vi "Compute Optimal Transition Time.vi"(8 "error in (no error)":errorcluster, 10 "optimum":T1, 11 "SV Square in":refnum<class "SV Square.lvclass">) -> (0 "error out":errorcluster, 2 "optimal transition time":dbl, 3 "SV Square out":refnum<class "SV Square.lvclass">)   [LabVIEW 2017, in "SV Square.lvclass"]
uses:
  <vilib>/addons/_NISVFA/_Generation/Signal Generation/SV Square/SV Square.lvclass
  C:/Program Files (x86)/National Instruments/LabVIEW 2017/vi.lib/addons/_NISVFA/_Generation/Signal Generation/SV Signal/SV Signal.lvclass
  C:/Program Files (x86)/National Instruments/LabVIEW 2017/vi.lib/addons/_NISVFA/_Generation/Signal Generation/SV Function/SV Function.lvclass
  <vilib>/addons/_NISVFA/_Generation/subVIs/sv_Optimum Location.ctl
  <vilib>/addons/_NISVFA/_Generation/Signal Generation/SV Signal/sv_Signal State Attribute.ctl
  <vilib>/addons/_NISVFA/_Generation/Signal Generation/SV Square/SV Square.lvclass/SV Square.ctl
  <vilib>/addons/_NISVFA/_Generation/Signal Generation/SV Signal/Read Sample Rate.vi
  <vilib>/addons/_NISVFA/_Generation/Signal Generation/SV Signal/SV Signal.lvclass
  <vilib>/addons/_NISVFA/_Generation/Signal Generation/SV Function/SV Function.lvclass
  <vilib>/addons/_NISVFA/_Generation/SoundVib_Generation.lvlib
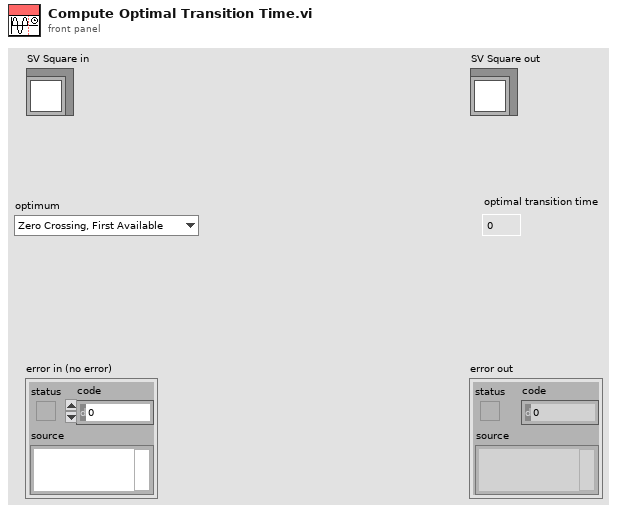
[diagram p1: front panel]
types:
  T1 = typedef "SoundVib_Generation.lvlib/sv_Optimum Location.ctl" = enum16{"Zero Crossing, First Available", "Zero Crossing, Positive Slope", "Zero Crossing, Negative Slope", "Peak or Valley", "Peak", "Valley"}
  T2 = typedef "SV Signal.lvclass/sv_Signal State Attribute.ctl" = string
  T3 = typedef "SV Signal.lvclass/sv_System Timing Model.ctl" = i64
  T4 = typedef "SV Signal.lvclass/sv_Generation State.ctl" = enum16{"Idle", "Ramp Up", "Pre-Measurement Settling", "Measurement", "Post-Measurement Settling", "Discrete Sweep Transition", "Ramp Down", "Update"}
  T5 = cluster{"system timing model":T3, "state":cluster{"RESET":bool, "generator timestamp":timestamp, "elapsed seconds":dbl, "elapsed samples":u64, "generation state":T4, "time offset at state":dbl, "samples generated at state":u64, "signal state":variant}, "duration of state":dbl, "samples remaining at state":i32}
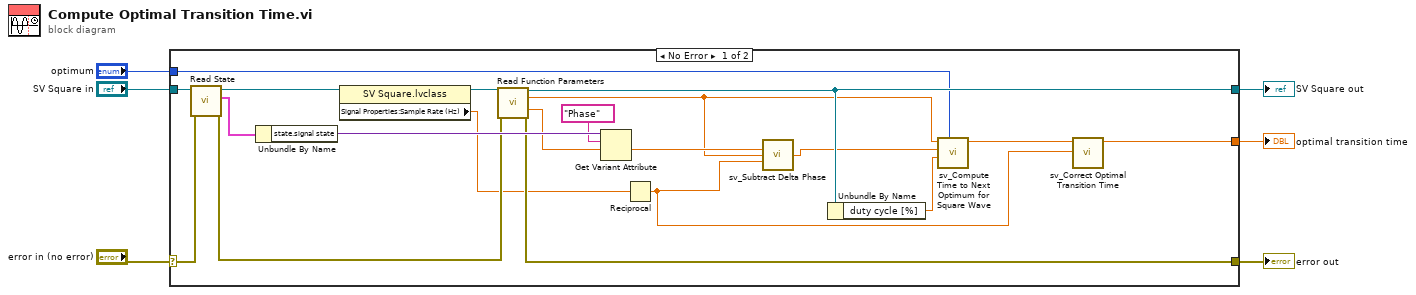
[diagram p0: block diagram]
diagram:
  n1 = case shown="No Error" "error in (no error)" {
    selector: "error in (no error)" -> [w25 w28]
    tunnel: [w16 w28] -> w5
    tunnel: "optimum" -> [w18 _]
    tunnel: [w20 w27] -> w3
    tunnel: "SV Square in" -> [w26 w27]
    tunnel: [w11 _] -> w1
    frame No Error {
      n2 = call <vilib>:"Read State.vi"("error in (no error)"=w25, "signal configuration"=w26) -> ("error out"=w17:errorcluster, "generator state"=w21:T5, "signal configuration"=w15:refnum<class "SV Square.lvclass">)  [unwired: 7 in]
      n3 = Unbundle By Name(w21) -> ("state.signal state"=w24:variant)
      n4 = property class="SV Square.lvclass"(reference=w15) -> (reference out=w14:refnum<class "SV Square.lvclass">, "Signal Properties:Sample Rate (Hz)"=w13:dbl)  [unwired: 1 in, 1 out]
      n5 = call <vilib>:"Read Function Parameters.vi"("signal configuration"=w14, "error in (no error)"=w17) -> ("signal configuration"=w20:refnum<class "SV Square.lvclass">, "frequency_Hz"=w8:dbl, "initial_phase_deg"=w22:dbl, "error out"=w16:errorcluster)  [unwired: 8 in, 2 out]
      n6 = Get Variant Attribute(Variant=w24, name=T2 "Phase", default value (empty Variant)=w22) -> (value=w10:dbl)  [unwired: 1 in, 3 out]
      n7 = Reciprocal(x=w13) -> (1/x=w7:dbl)
      n8 = call <vilib>:"sv_Subtract Delta Phase.vi"("phase in [deg]"=w10, "frequency [Hz]"=w8, "dt [s]"=w7) -> ("phase out [deg]"=w9:dbl)  [unwired: 12 in]
      n9 = Unbundle By Name(w20) -> ("duty cycle [%]"=w19:dbl)
      n10 = call <vilib>:"sv_Compute Time to Next Optimum for Square Wave.vi"("optimum"=w18, "duty cycle (50 %)"=w19, "phase (0 °)"=w9, "frequency (997 Hz)"=w8) -> ("time to optimum [s]"=w12:dbl)  [unwired: 7 in]
      n11 = call <vilib>:"sv_Correct Optimal Transition Time.vi"("dt"=w7, "time to optimum [s]"=w12) -> ("corrected time to optimum [s]"=w11:dbl)  [unwired: 9 in]
    }
    frame Error {
    }
  }
  "error out" <- w5
  "SV Square out" <- w3
  "optimal transition time" <- w1
